vi "get file names.vi"() -> (2 "UDP data filenames":string[](array[string]))   [LabVIEW 2021]
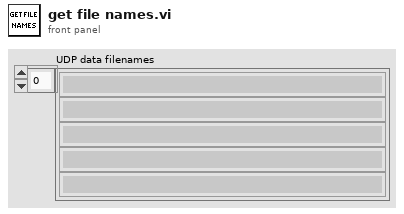
[diagram p1: front panel]
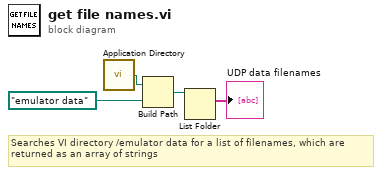
[diagram p0: block diagram]
diagram:
  # "Searches VI directory /emulator data for a list of filenames, which are\nreturned as an array of strings"
  n1 = call <vilib>:"Application Directory.vi"() -> ("Application Directory"=w4:path)
  n2 = Build Path(base path=w4, name or relative path=path "emulator data") -> (appended path=w2:path)
  n3 = List Folder(path=w2) -> (filenames=→"UDP data filenames":string[])  [unwired: 3 in, 3 out]
